vi "victrl.vi"   [LabVIEW 2012]
doc: "The victrl.vi CGI can be used to set Boolean, numeric and string control values of any running VI. It can also be used to open and close panels of other VIs and to set VIs running. See /examples/victrlpr.htm for more information."
uses:
  <vilib>/addons/internet/NI_InternetTK_Core_VIs.lvlib
  <vilib>/addons/internet/NI_InternetTK_Common_VIs.lvlib
types:
  T1 = typedef "CGI Connection Info.ctl" = cluster{"name":string, "type":T2, "session":T3}
  T2 = typedef "CGI Request Type.ctl" = enum16{"cgi", ".spool first", ".spool", ".spool last"}
  T3 = typedef "HTTP Session.ctl" = refnum<k1>
  T4 = typedef "NI_FTP.lvlib/Keyed Array.ctl" = cluster{"keys":string[], "values":string[]}
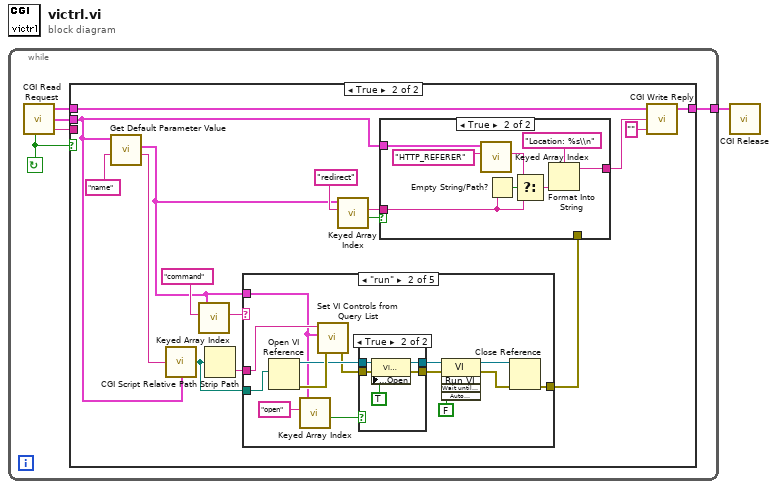
[diagram p0: block diagram]
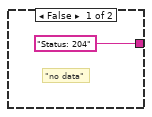
[diagram p3: hidden frame]
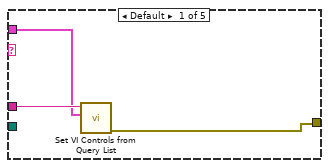
[diagram p4: hidden frame]
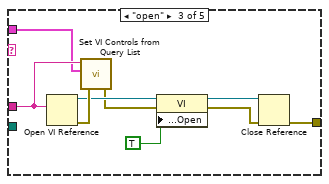
[diagram p6: hidden frame]
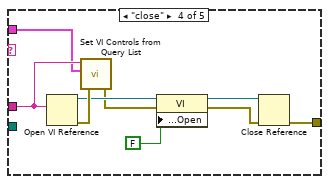
[diagram p7: hidden frame]
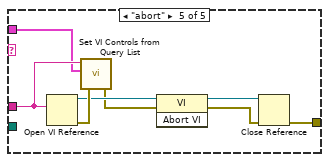
[diagram p8: hidden frame]
diagram:
  n1 = while {
    tunnel: [w5] -> w1
    stop <- w4 continue-if-true
    n2 = call <vilib>:"CGI Read Request.vi"() -> ("valid request?"=w4:bool, "cgi connection info"=w6:T1, "env"=w3:T4, "content"=w2:string)  [unwired: 4 in]
    n3 = case shown="True" w4 {
      tunnel: [w7 w23] -> w5
      tunnel: w6 -> [w7 w22]
      tunnel: w3 -> [_ w14]
      tunnel: w2 -> [_ _]
      frame False {
      }
      frame True {
        n4 = call "Get Default Parameter Value.vi"("default param name"="name" ("key"), "env"=w14) -> ("default param value"=w10:string, "query"=w12:T4)  [unwired: 2 in, 2 out]
        n5 = call <vilib>:"CGI Script Relative Path.vi"("relative unix path"=w10, "env"=w14) -> ("absolute path"=w9:path)
        n6 = call <vilib>:"Keyed Array Index.vi"("key"="command", "array in"=w12) -> ("value"=w13:string)  [unwired: 3 in, 2 out]
        n7 = Strip Path(path=w9) -> (name=w20:string)  [unwired: 1 out]
        n8 = case shown="\"run\"" w13 {
          tunnel: w12 -> [w34 w43 w63 w72 w80]
          tunnel: w9 -> [_ w45 _ _ _]
          tunnel: w20 -> [w35 w48 w64 w73 w81]
          tunnel: [w33 w36 w57 w66 w75] -> w8
          frame Default {
            n9 = call "Set VI Controls from Query List.vi"("query params"=w34, "name"=w35) -> ("error out"=w33:errorcluster)  [unwired: 5 in]
          }
          frame "run" {
            n10 = Open VI Reference(vi path=w45) -> (vi reference=w47:refnum<vi>, error out=w49:errorcluster)  [unwired: 5 in]
            n11 = call <vilib>:"Keyed Array Index.vi"("key"="open", "array in"=w43) -> ("valid key"=w42:bool)  [unwired: 3 in, 2 out]
            n12 = call "Set VI Controls from Query List.vi"("error in (no error)"=w49, "query params"=w43, "name"=w48) -> ("error out"=w46:errorcluster)  [unwired: 4 in]
            n13 = case shown="True" w42 {
              tunnel: w47 -> [w51 w56]
              tunnel: w46 -> [w50 w55]
              tunnel: [w51 w53] -> w41
              tunnel: [w50 w52] -> w40
              frame False {
              }
              frame True {
                n14 = property class="VirtualInstrument"(reference=w56, error in=w55, "Front Panel Window:Open"=TRUE ("Front Panel.Open")) -> (reference out=w53:refnum<vi>, error out=w52:errorcluster)
              }
            }
            n15 = invoke class="VI" method="Run VI"(reference=w41, error in=w40, "Wait until done"=FALSE) -> (reference out=w37:refnum<vi>, error out=w38:errorcluster)  [unwired: 2 in, 3 out]
            n16 = Close Reference(reference=w37, error in (no error)=w38) -> (error out=w36:errorcluster)
          }
          frame "open" {
            n17 = Open VI Reference(vi path=w64) -> (vi reference=w62:refnum<vi>, error out=w65:errorcluster)  [unwired: 5 in]
            n18 = call "Set VI Controls from Query List.vi"("error in (no error)"=w65, "query params"=w63, "name"=w64) -> ("error out"=w61:errorcluster)  [unwired: 4 in]
            n19 = property class="VI"(reference=w62, error in=w61, "Front Panel Window:Open"=TRUE ("Front Panel.Open")) -> (reference out=w59:refnum<vi>, error out=w58:errorcluster)
            n20 = Close Reference(reference=w59, error in (no error)=w58) -> (error out=w57:errorcluster)
          }
          frame "close" {
            n21 = Open VI Reference(vi path=w73) -> (vi reference=w71:refnum<vi>, error out=w74:errorcluster)  [unwired: 5 in]
            n22 = call "Set VI Controls from Query List.vi"("error in (no error)"=w74, "query params"=w72, "name"=w73) -> ("error out"=w70:errorcluster)  [unwired: 4 in]
            n23 = property class="VI"(reference=w71, error in=w70, "Front Panel Window:Open"=FALSE ("Front Panel.Open")) -> (reference out=w68:refnum<vi>, error out=w67:errorcluster)
            n24 = Close Reference(reference=w68, error in (no error)=w67) -> (error out=w66:errorcluster)
          }
          frame "abort" {
            n25 = Open VI Reference(vi path=w81) -> (vi reference=w79:refnum<vi>, error out=w82:errorcluster)  [unwired: 5 in]
            n26 = call "Set VI Controls from Query List.vi"("error in (no error)"=w82, "query params"=w80, "name"=w81) -> ("error out"=w78:errorcluster)  [unwired: 4 in]
            n27 = invoke class="VI" method="Abort VI"(reference=w79, error in=w78) -> (reference out=w77:refnum<vi>, error out=w76:errorcluster)  [unwired: 1 in, 1 out]
            n28 = Close Reference(reference=w77, error in (no error)=w76) -> (error out=w75:errorcluster)
          }
        }
        n29 = call <vilib>:"Keyed Array Index.vi"("key"="redirect", "array in"=w12) -> ("valid key"=w18:bool, "value"=w17:string)  [unwired: 3 in, 1 out]
        n30 = case shown="True" w18 {
          tunnel: w17 -> [_ w29]
          tunnel: ["Status: 204" w31] -> w16
          tunnel: w14 -> [_ w25]
          tunnel: w8 -> [_ _]
          frame False {
            # "\"no data\""
          }
          frame True {
            n31 = call <vilib>:"Keyed Array Index.vi"("key"="HTTP_REFERER", "array in"=w25) -> ("value"=w26:string)  [unwired: 3 in, 2 out]
            n32 = Empty String/Path?(string/path=w29) -> (empty?=w30:bool)
            n33 = Select(t=w26, s=w30, f=w29) -> (s? t:f=w28:string)
            n34 = Format Into String(format string="Location: %s\\n", w28) -> (resulting string=w31:string)  [unwired: 2 in, 1 out]
          }
        }
        n35 = call <vilib>:"CGI Write Reply.vi"("content"="", "header"=w16, "cgi connection info"=w22) -> ("cgi connection info out"=w23:T1)  [unwired: 2 in]
      }
    }
  }
  n36 = call <vilib>:"CGI Release.vi"("cgi connection info"=w1) -> ()  [unwired: 5 in]
